vi "Spectrum.vi"(0 "Spectrum Parameters":T2={"Window 1 time (s)"=2e-05, "Window 2 time (s)"=1e-06, "Window 3 time (s) "=5e-08, "Window 4 time (s)"=2e-06, "Path to SpectrumBurn"=path "C:/Users/Loncar/Desktop/ESR VIs - Srujan/Sam Kim/PB/ESRFreq.exe", "Window 5 time (s)"=1e-07, "Window 6 time (s)"=5e-08, "Window 1 active channels"=[FALSE, TRUE], "Window 2 active channels"=[], "Window 3 active channels "=[FALSE, FALSE, TRUE], "Window 4 active channels"=[TRUE, FALSE, TRUE], "Window 5 active channels"=[FALSE, FALSE, TRUE], "Window 6 active channels"=[]}, 1 "Optimize Parameters":T1={"Volt Step"={"X"=0.01, "Y"=0.01, "Z"=0.0}, "Num Iterations"=1, "Dwell Time (ms)"=100, "Volts Range"={"X"=0.1, "Y"=0.1, "Z"=0.0}, "Method"={"X"=enum."Max", "Y"=enum."Max"}} {"Volts Range"."Z" min=0.0; "Volts Range"."Y" min=0.0; "Volts Range"."X" min=0.0; "Dwell Time (ms)" min=0; "Num Iterations" min=1 step=1; "Volt Step"."Z" min=0.0; "Volt Step"."Y" min=1e-06; "Volt Step"."X" min=1e-06}, 2 "Num Scan Iterations":i32, 3 "V min":dbl=-0.3, 4 "V max":dbl=0.3, 5 "# V steps":dbl, 6 "Save 2D counts array to spreadsheet?":bool, 7 "# Samples per laser voltage point":i32, 8 "Path for 2D counts spreadsheet":path=path "C:/experiment/data/may_15_2012/SIL1_NV1_pippin_uW_off", 9 "Counts vs laser IntGraph Refnum":refnum<vi>, 10 "Save intensity graph?":bool, 11 "Pict Refnum":refnum<vi>, 12 "Path for intensity graph":path=path "C:/experiment/data/may_15_2012/SIL1_NV1_pippin_uW_off", 14 "Save avg counts data to spreadsheet?":bool, 15 "Path for avg spectrum spreadsheet":path=path "C:/experiment/data/may_15_2012/SIL1_NV1_pippin_uW_off", 16 "Save avg spectrum graph?":bool, 17 "Path for avg spectrum graph":path=path "C:/experiment/data/may_15_2012/SIL1_NV1_pippin_uW_off") -> ()   [LabVIEW 2012]
uses:
  <vilib>/Analysis/NI_AALBase.lvlib
  <vilib>/Utility/file.llb/Write To Spreadsheet File (DBL).vi
  Channels.vi
  <vilib>/DAQmx/read.llb/DAQmx Read (Counter 1D U32 1Chan NSamp).vi
  <vilib>/Analysis/baseanly.llb/Mean (DBL).vi
  Global Vars.vi
  Spectrum Window Parameters.ctl
  Strict Type Def - Optimize Parameters Cluster.ctl
panel:
  out "Average counts":picture
  out "Counts vs. laser voltage":u32[][](graph)
  out "2D array of # counts":u32[][](array[numeric])
  # "VI for (single shot) resonance fluorescence spectroscopy\nDated: 05/27/2013"
  # "Window descriptions and states of PB signals:\n1. Green AOM on\n2. All off\n3. Counter sample clk on\n4. Red AOM on, counter sample clk on\n5. Counter sample clk on\n6. All off\n\nConsidering AOM delay, try making the foll changes:\n1. Green AOM on - few us (take turn-on time into consideration)\n2. Red AOM on - 0.75 us (during this window, green AOM turns off and red AOM turns on)\n3. Red AOM on, counter sample clk on - custom\n4. Counter sample clk on - 0.75 us (during this period red AOM turns off)"
  # "Default PB connections:\nPB0 - Red AOM\nPB1 - Green AOM\nPB2 - Counter sample clk"
  # "Laser Set:"
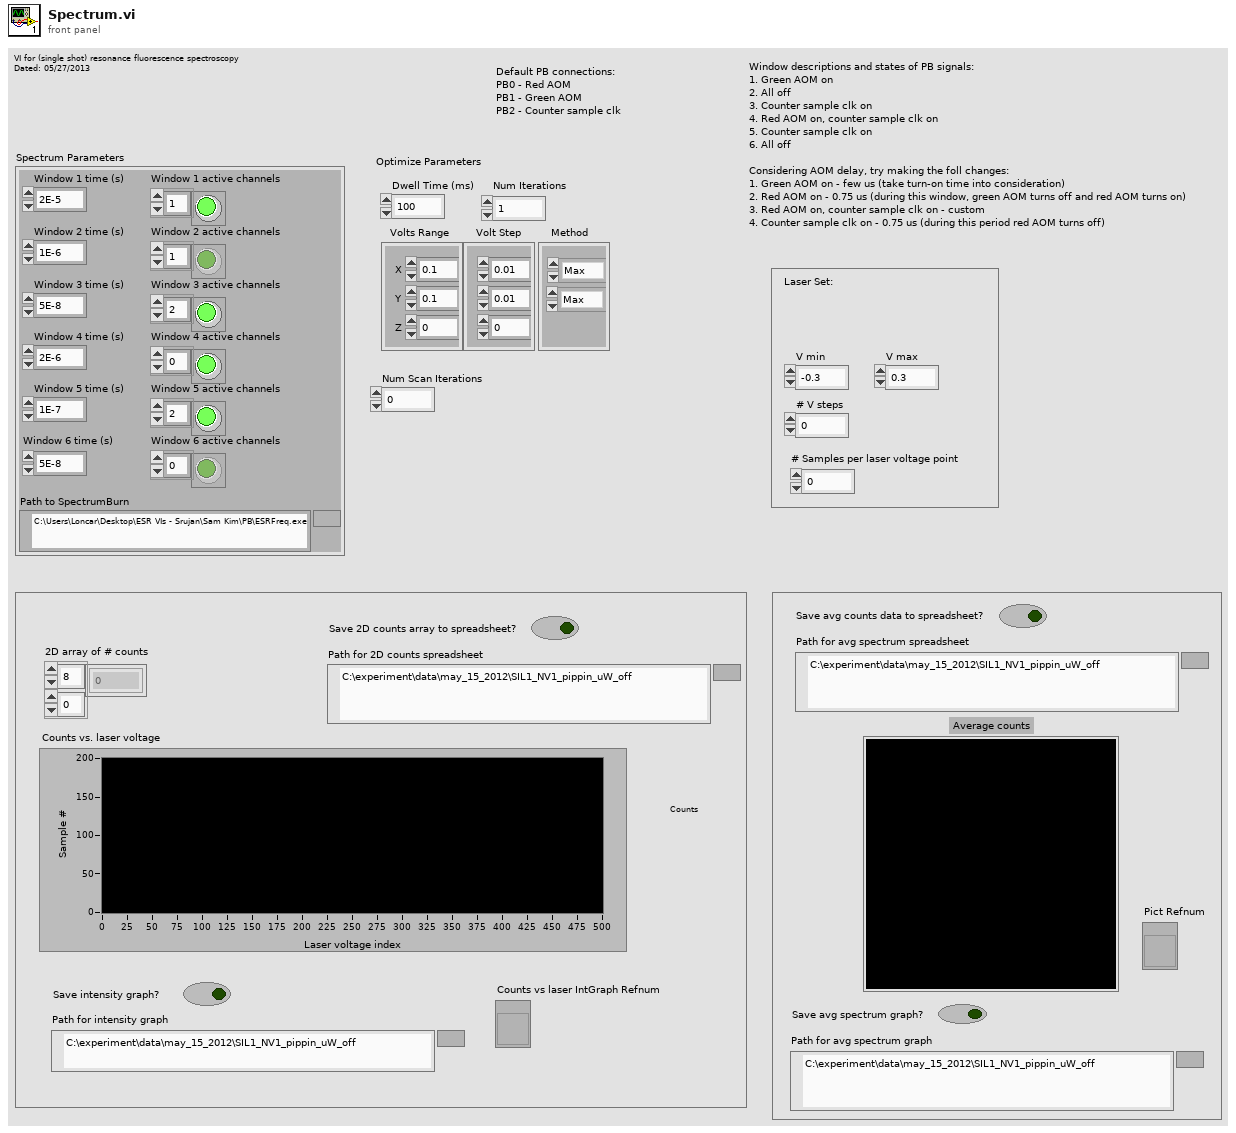
[diagram p1: front panel]
types:
  T1 = typedef "Strict Type Def - Optimize Parameters Cluster.ctl" = cluster{"Volt Step":cluster{"X":dbl, "Y":dbl, "Z":dbl}, "Num Iterations":i32, "Dwell Time (ms)":i32, "Volts Range":cluster{"X":dbl, "Y":dbl, "Z":dbl}, "Method":cluster{"X":enum16{"Max", "Gaussian"}, "Y":enum16{"Max", "Gaussian"}}}
  T2 = typedef "Spectrum Window Parameters.ctl" = cluster{"Window 1 time (s)":dbl, "Window 2 time (s)":dbl, "Window 3 time (s) ":dbl, "Window 4 time (s)":dbl, "Path to SpectrumBurn":path, "Window 5 time (s)":dbl, "Window 6 time (s)":dbl, "Window 1 active channels":bool[], "Window 2 active channels":bool[], "Window 3 active channels ":bool[], "Window 4 active channels":bool[], "Window 5 active channels":bool[], "Window 6 active channels":bool[]}
  T3 = typedef "imagedata.ctl" = cluster{"image type":i32, "image depth":i32, "image":u8[], "mask":u8[], "colors":u32[], "Rectangle":cluster{"left":i16, "top":i16, "right":i16, "bottom":i16}}
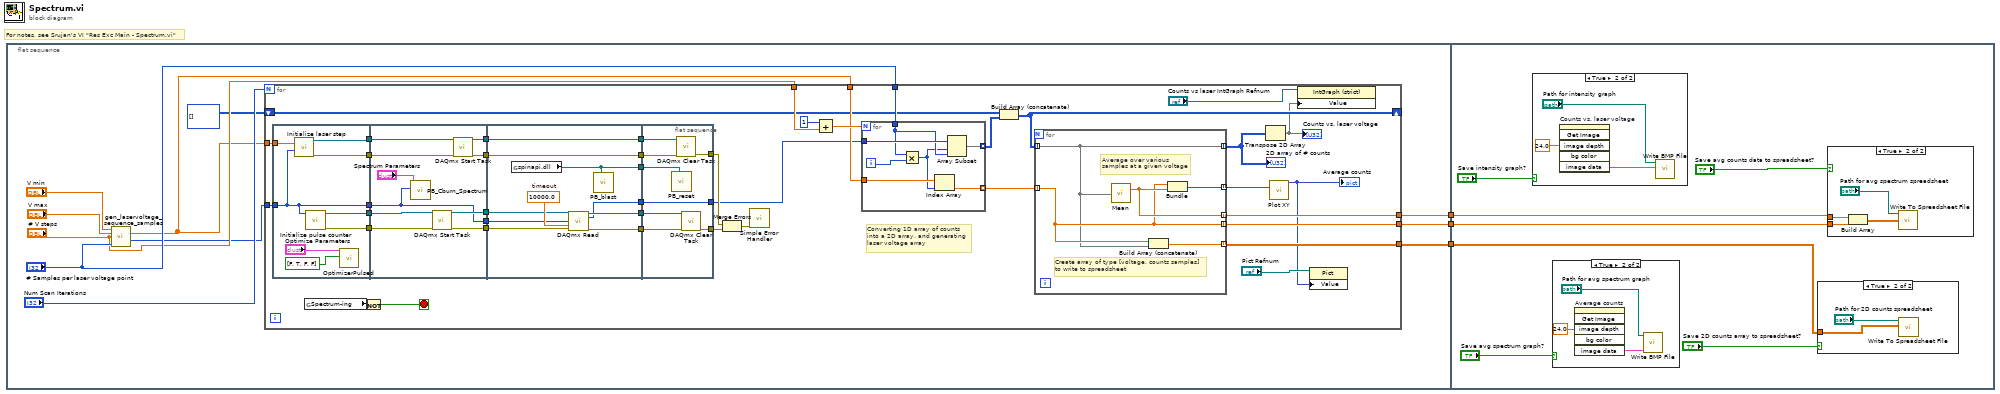
[diagram p0: block diagram]
diagram:
  # "For notes, see Srujan's VI \"Res Exc Main - Spectrum.vi\""
  n1 = flat-sequence {
    tunnel: [w14] -> w3
    tunnel: [w13] -> w2
    tunnel: [w12] -> w1
    tunnel: w3 -> [w108]
    tunnel: w2 -> [w105]
    tunnel: w1 -> [w106]
    frame #0 {
      n2 = call "gen_laservoltage_sequence_samples.vi"("V min"="V min", "V max"="V max", "# V steps"="# V steps", "# Samples per voltage point"="# Samples per laser voltage point") -> ("Voltage sequence"=w5:dbl[], "Total # data points"=w4:i32)  [unwired: 10 in]
      n3 = for {
        N: "Num Scan Iterations" -> [_]
        tunnel: [w39] -> w14
        tunnel: [w38] -> w13
        tunnel: [w37] -> w12
        tunnel: "# Samples per laser voltage point" -> [w34]
        tunnel: "# V steps" -> [w33]
        tunnel: w5 -> [w30]
        tunnel: w4 -> [w27]
        shift-right: [w22] -> _
        shift-left: i32[][] [] ("Flourescence Data") -> [w24]
        tunnel: w5 -> [w21]
        stop <- w19 stop-if-true
        # "Converting 1D array of counts \ninto a 2D array, and generating \nlaser voltage array"
        n4 = flat-sequence {
          tunnel: w27 -> [w64]
          tunnel: [w64] -> w56
          tunnel: [w67] -> w55
          tunnel: [w66] -> w54
          tunnel: [w69] -> w53
          tunnel: [w68] -> w52
          tunnel: w21 -> [w65]
          tunnel: [w81] -> w51
          tunnel: [w80] -> w50
          tunnel: [w77] -> w49
          tunnel: [w76] -> w48
          tunnel: [w74] -> w47
          tunnel: w56 -> [w74]
          tunnel: w55 -> [w79]
          tunnel: w54 -> [w78]
          tunnel: w53 -> [w73]
          tunnel: w52 -> [w72]
          tunnel: w51 -> [w90]
          tunnel: w50 -> [w89]
          tunnel: [w84] -> w46
          tunnel: [w88] -> w45
          tunnel: [w87] -> w44
          tunnel: [w86] -> w43
          tunnel: w49 -> [w86]
          tunnel: w48 -> [w85]
          tunnel: [w85] -> w42
          tunnel: w47 -> [w83]
          tunnel: [w82] -> w41
          tunnel: [w99] -> w25
          tunnel: w46 -> [w99]
          tunnel: w45 -> [w98]
          tunnel: w44 -> [w97]
          tunnel: w43 -> [w94]
          tunnel: w42 -> [w93]
          tunnel: [w96] -> w36
          tunnel: w41 -> [w95]
          tunnel: [w92] -> w26
          frame #0 {
            n5 = call "Initialize laser step.vi"("Total # data points"=w64, "Voltage sequence"=w65) -> ("error out"=w66:errorcluster, "Task out"=w67:refnum<k21>)  [unwired: 8 in]
            n6 = call "Initialize pulse counter.vi"("Samples per channel"=w64) -> ("error out"=w68:errorcluster, "DAQmx Task Name"=w69:refnum<k21>)  [unwired: 9 in]
            n7 = call "OptimizerPulsed.vi"("Optimize active channels"=bool[] [FALSE, TRUE, FALSE, FALSE], "Optimize Parameters"="Optimize Parameters") -> ()  [unwired: 9 in, 1 out]
          }
          frame #1 {
            n8 = call "PB_Cburn_Spectrum.vi"("Spectrum Parameters"="Spectrum Parameters", "# scans before track"=w74) -> ()  [unwired: 8 in, 1 out]
            n9 = call <vilib>:"DAQmx Start Task.vi"("task/channels in"=w73, "error in"=w72) -> ("task out"=w81:refnum<k21>, "error out"=w80:errorcluster)  [unwired: 12 in]
            n10 = call <vilib>:"DAQmx Start Task.vi"("task/channels in"=w79, "error in"=w78) -> ("task out"=w77:refnum<k21>, "error out"=w76:errorcluster)  [unwired: 12 in]
          }
          frame #2 {
            w91 = 10000.0  # timeout
            n11 = global read "Channels.vi" "spinapi.dll"() -> (w82:path)
            n12 = call-poly <vilib>:"DAQmx Read.vi"("task/channels in"=w90, "number of samples per channel"=w83, "timeout"=w91, "error in"=w89) -> ("task out"=w87:refnum<k21>, "data"=w84:u32[], "error out"=w88:errorcluster)  [unwired: 9 in]
            n13 = call "PB_blast.vi"("Path to spinapi.dll"=w82) -> ()  [unwired: 7 in]
          }
          frame #3 {
            n14 = call "PB_reset.vi"("Path to spinapi.dll"=w95) -> ()  [unwired: 7 in]
            n15 = call <vilib>:"DAQmx Clear Task.vi"("task in"=w94, "error in"=w93) -> ("error out"=w92:errorcluster)  [unwired: 13 in]
            n16 = call <vilib>:"DAQmx Clear Task.vi"("task in"=w97, "error in"=w98) -> ("error out"=w96:errorcluster)  [unwired: 13 in]
          }
        }
        n17 = global read "Global Vars.vi" "Spectrum-ing"() -> (w20:bool)
        n18 = Not(x=w20) -> (.not. x?=w19:bool)
        n19 = Merge Errors(w26, w36) -> (w35:errorcluster)
        n20 = call <vilib>:"Simple Error Handler.vi"("error in (no error)"=w35) -> ()  [unwired: 4 in, 5 out]
        n21 = Add(x=1, y=w33) -> (x+y=w31:dbl)
        n22 = for {
          N: w31 -> [_]
          tunnel: w25 -> [w63]
          tunnel: w34 -> [w62]
          tunnel: [w61] -> w23 mode=indexing
          tunnel: w30 -> [w59]
          tunnel: [w57] -> w29 mode=indexing
          i -> [w60]
          n23 = Multiply(x=w62, y=w60) -> (x*y=w58:i32)
          n24 = Index Array(array=w59, index=w58) -> (element=w57:dbl)
          n25 = Array Subset(array=w63, index=w58, length=w62) -> (w61:u32[])
        }
        n26 = Build Array (concatenate)(w24, w23) -> (w22:u32[][])
        n27 = for {
          tunnel: [w101] -> w40 mode=indexing
          tunnel: [w102] -> w39 mode=indexing
          tunnel: [w104] -> w38 mode=indexing
          tunnel: [w103] -> w37 mode=indexing
          tunnel: w29 -> [w102] mode=indexing
          tunnel: w22 -> [w101] mode=indexing
          tunnel: [w100] -> w28 mode=indexing
          # "Create array of type [voltage, counts samples]\nto write to spreadsheet"
          # "Average over various \nsamples at a given voltage"
          n28 = call-poly <vilib>:"Mean.vi"("X"=w101) -> ("mean"=w104:dbl)  [unwired: 1 out]
          n29 = Build Array (concatenate)(w102, w101) -> (w103:dbl[])
          n30 = Bundle("element"=w102, "mean"=w104) -> (w100:cluster{"element":dbl, "mean":dbl})  [unwired: 1 in]
        }
        "2D array of # counts" <- w40
        n31 = Transpose 2D Array(2D array=w40) -> (transposed array=w17:u32[][])
        "Counts vs. laser voltage" <- w17
        n32 = call <vilib>:"Plot XY.vi"("data"=w28) -> ("new picture"=w15:picture)  [unwired: 14 in]
        "Average counts" <- w15
        n33 = property class="IntGraph (strict)"(reference="Counts vs laser IntGraph Refnum", "Value"=w17) -> ()  [unwired: 1 in, 2 out]
        n34 = property class="Pict"(reference="Pict Refnum", "Value"=w15) -> ()  [unwired: 1 in, 2 out]
      }
    }
    frame #1 {
      n35 = case shown="True" "Save intensity graph?" {
        frame False {
        }
        frame True {
          n36 = invoke on="Counts vs. laser voltage" class="IntGraph (strict)" method="Get Image"("image depth"=24.0 ("Initial Delay")) -> ("image data"=w123:T3)  [unwired: 5 in, 5 out]
          n37 = call <vilib>:"Write BMP File.vi"("image data"=w123, "path to BMP file"="Path for intensity graph") -> ()  [unwired: 8 in, 2 out]
        }
      }
      n38 = case shown="True" "Save avg spectrum graph?" {
        frame False {
        }
        frame True {
          n39 = invoke on="Average counts" class="Pict" method="Get Image"("image depth"=24.0 ("Initial Delay")) -> ("image data"=w118:T3)  [unwired: 5 in, 5 out]
          n40 = call <vilib>:"Write BMP File.vi"("image data"=w118, "path to BMP file"="Path for avg spectrum graph") -> ()  [unwired: 8 in, 2 out]
        }
      }
      n41 = case shown="True" "Save 2D counts array to spreadsheet?" {
        tunnel: w106 -> [_ w112]
        frame False {
        }
        frame True {
          n42 = call-poly <vilib>:"Write To Spreadsheet File.vi"("2D data"=w112, "file path (dialog if empty)"="Path for 2D counts spreadsheet") -> ()  [unwired: 6 in, 1 out]
        }
      }
      n43 = case shown="True" "Save avg counts data to spreadsheet?" {
        tunnel: w108 -> [_ w115]
        tunnel: w105 -> [_ w116]
        frame False {
        }
        frame True {
          n44 = Build Array(w116, w115) -> (w114:dbl[][])
          n45 = call-poly <vilib>:"Write To Spreadsheet File.vi"("2D data"=w114, "file path (dialog if empty)"="Path for avg spectrum spreadsheet") -> ()  [unwired: 6 in, 1 out]
        }
      }
    }
  }
